vi "detChecksum.vi"(8 "error in (no error)":errorcluster, 10 "inputString":string, 11 "EncoderReader in":refnum<class "EncoderReader.lvclass">) -> (0 "error out":errorcluster, 2 "checksumString":string, 3 "EncoderReader out":refnum<class "EncoderReader.lvclass">)   [LabVIEW 2013, in "EncoderReader.lvclass"]
uses:
  EncoderReader.lvclass
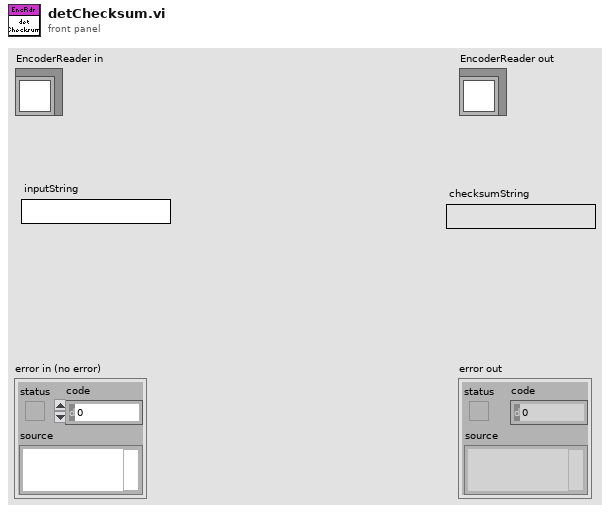
[diagram p1: front panel]
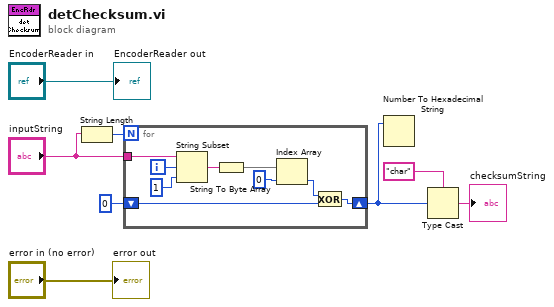
[diagram p0: block diagram]
diagram:
  n1 = String Length(string="inputString") -> (length=w5:i32)
  n2 = for {
    N: w5 -> [_]
    tunnel: "inputString" -> [w17]
    shift-right: [w10] -> w3
    shift-left: u8 0 -> [w9]
    i -> [w16]
    n3 = String Subset(string=w17, offset (0)=w16, length (rest)=1) -> (substring=w14:string)
    n4 = String To Byte Array(string=w14) -> (unsigned byte array=w11:u8[])
    n5 = Index Array(array=w11, index=0) -> (element=w13:u8)
    n6 = Exclusive Or(1:w9, 2:w13) -> (0:w10:u8)
  }
  n7 = Number To Hexadecimal String(2:w3) -> ()  [unwired: 2 out]
  n8 = Type Cast(type="char", x=w3) -> (*(type *) &x=→"checksumString":string)
  "error out" <- "error in (no error)"
  "EncoderReader out" <- "EncoderReader in"
